vi "DB_GetPath.vi"() -> (3 "appended path":path)   [LabVIEW 2015, in "Settings-Style.lvlib"]
uses:
  Settings-Style.lvlib
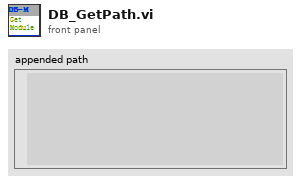
[diagram p1: front panel]
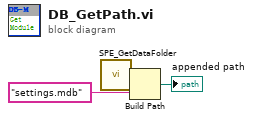
[diagram p0: block diagram]
diagram:
  n1 = call "SPE_GetDataFolder.vi"() -> ("data folder path"=w1:path)  [unwired: 15 in]
  n2 = Build Path(base path=w1, name or relative path="settings.mdb") -> (appended path=→"appended path":path)
